vi "Wait and Switch.vi"(8 "error in":errorcluster, 9 "Wait for":dbl[unit], 10 "Switch to":bool, 11 "task in":refnum<k21>) -> (0 "error out":errorcluster, 3 "task out":refnum<k21>)   [LabVIEW 2017]
uses:
  <vilib>/DAQmx/write.llb/DAQmx Write (Digital Bool 1Line 1Point).vi
  <vilib>/DAQmx/miscellaneous.llb/DAQmx Fill In Error Info.vi
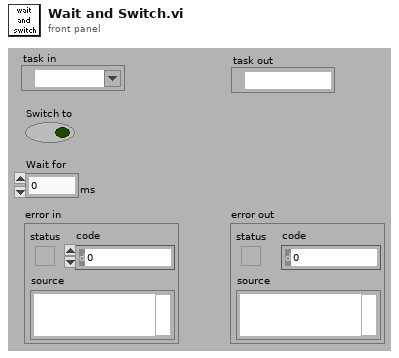
[diagram p1: front panel]
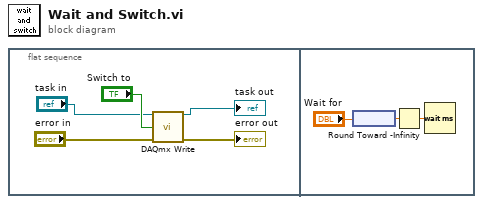
[diagram p0: block diagram]
diagram:
  n1 = flat-sequence {
    frame #0 {
      n2 = call-poly <vilib>:"DAQmx Write.vi"("task/channels in"="task in", "data"="Switch to", "error in"="error in") -> ("task out"=→"task out":refnum<k21>, "error out"=→"error out":errorcluster)  [unwired: 1 in, 10 out]
    }
    frame #1 {
      n3 = node("Wait for") -> (w7:dbl)
      n4 = Round Toward -Infinity(1:w7) -> (0:w6:dbl)
      n5 = Wait (ms)(milliseconds to wait=w6) -> ()  [unwired: 1 out]
    }
  }
